vi "Dashboard Main.vi"() -> ()   [LabVIEW 2011]
uses:
  Dashboard Datatype.ctl
  <vilib>/Rock Robotics/WPI/DriverStation/WPI_DriverStationDigitalData.ctl
  <vilib>/vision/NI_Vision_Development_Module.lvlib
panel:
  out "Bounding Box":T1
  out "TargetDistance":dbl
  out "Camera Image 2":T2(plugin-control) caption="Zoomed Image"
  out "Odometer":dbl
  out "Encoders":cluster{"Left Encoder":dbl, "Right Encoder":dbl}
  out "Launcher Rate":dbl
  out "Gyro":cluster{"Robot Gyro":dbl, "Robot Gyro":dbl}(knob) scale=-180.0..180.0
  out "8 -- Battery":sgl(graph)
  out "Analog Input":sgl[](array[slide]) scale=0.0..5.0
  in  "Viewer":enum32{"Camera Image", "Kinect Skeleton"}(tab)
  in  "Video Enable":bool=TRUE
  out "Camera Image":T2(plugin-control)
  out "Buttons 1":cluster{"1":bool, "2":bool, "3":bool}
  out "Kinect 1":cluster{"X":dbl, "Y":dbl, "Z":dbl} {"X" scale=1.0..-1.0; "Y" scale=1.0..-1.0; "Z" scale=1.0..-1.0}
  out "Buttons 2":cluster{"1":bool, "2":bool, "3":bool}
  out "Kinect 2":cluster{"X":dbl, "Y":dbl, "Z":dbl} {"X" scale=1.0..-1.0; "Y" scale=1.0..-1.0; "Z" scale=1.0..-1.0}
  out "Version":string
  out "Skeleton Picture":picture
  out "Players":i8
  out "Dashboard Datatype Warning":string="Warning: The Dashboard Datatype used by the robot project and this dashboard do not match.\nSee diagram for more details."
  out "Robot IP Address":string
  out "Image Error Message":string="Timeout in Camera Communications"
  out "Solenoid Output":bool[](array[boolean])
  out "PWM":cluster{u8, u8}[](array[slide])=[{0, 157}, {0, 157}, {0, 157}, {0, 157}, {0, 157}, {0, 157}, {0, 157}, {0, 157}, {0, 157}, {0, 169}] scale=1.0..255.0
  out "GPIO Output Enable":bool[](array[boolean])
  out "GPIO State":bool[](array[boolean])
  out "Relay":cluster{"Forward":bool[], "Reverse":bool[]}
  # "Analog #1"
  # "1"
  # "7"
  # "Communications"
  # "Solenoid #1"
  # "1"
  # "8"
  # "Digital #1"
  # "1"
  # "10"
  # "1"
  # "14"
  # "1"
  # "8"
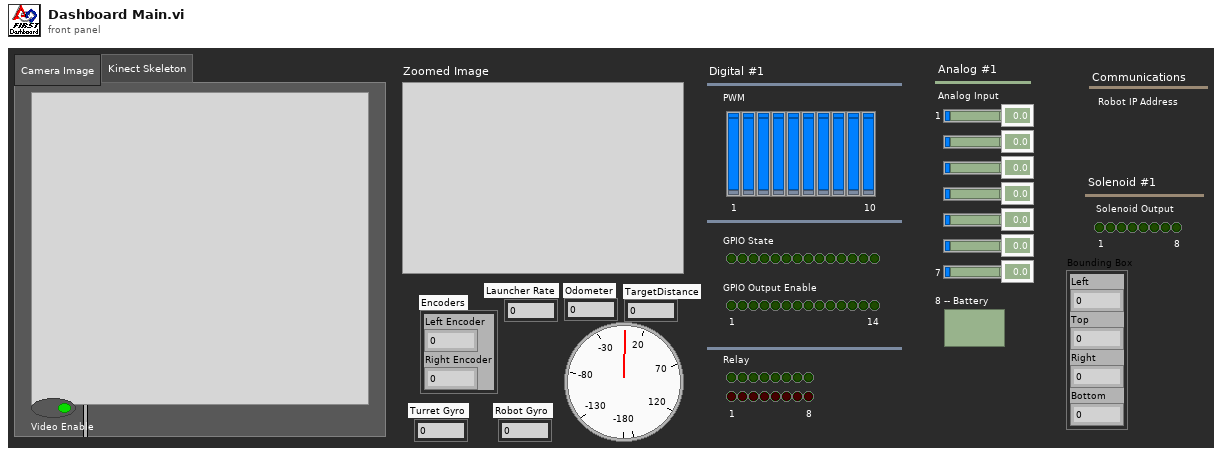
[diagram p1: front panel]
types:
  T1 = cluster{"Left":dbl, "Top":dbl, "Right":dbl, "Bottom":dbl}
  T2 = typedef "IMAQ Image.ctl" = refnum<image>
  T3 = typedef "Image Type" = u32
  T4 = typedef "Dashboard Datatype.ctl" = cluster{cluster{"AnalogModule[0]":cluster{"Channel[0]":sgl, "Channel[1]":sgl, "Channel[2]":sgl, "Channel[3]":sgl, "Channel[4]":sgl, "Channel[5]":sgl, "Channel[6]":sgl, "Channel[7]":sgl}, "AnalogModule[1]":cluster{"Channel[0]":sgl, "Channel[1]":sgl, "Channel[2]":sgl, "Channel[3]":sgl, "Channel[4]":sgl, "Channel[5]":sgl, "Channel[6]":sgl, "Channel[7]":sgl}}, cluster{"DigitalModule[0]":T5, "DigitalModule[1]":T5}, "Solenoid":u8, "Launcher Rate":dbl, "Gyros":cluster{"Turret Gyro":dbl, "Robot Gyro":dbl}, "Encoders":cluster{"Left Encoder":dbl, "Right Encoder":dbl}, "Drive Distance":dbl, "Bounding Box":cluster{"Left":dbl, "Top":dbl, "Right":dbl, "Bottom":dbl}, "Target Distance":dbl}
  T5 = typedef "WPI_DriverStationDigitalData.ctl" = cluster{"Relay Fwd":u8, "Relay Rev":u8, "GPIO":u16, "GPIO_OE":u16, "PWM":cluster{"PWM[0]":u8, "PWM[1]":u8, "PWM[2]":u8, "PWM[3]":u8, "PWM[4]":u8, "PWM[5]":u8, "PWM[6]":u8, "PWM[7]":u8, "PWM[8]":u8, "PWM[9]":u8}}
  T6 = cluster{cluster{"Left":dbl, "Bottom":dbl}, cluster{"Right":dbl, "Bottom":dbl}, cluster{"Right":dbl, "Top":dbl}, cluster{"Left":dbl, "Top":dbl}}
  T7 = typedef "LVRectTypeDef.ctl" = cluster{"left":i16, "top":i16, "right":i16, "bottom":i16}
  T8 = typedef "SkeletonTrackState.ctl" = enum32{"NotTracked", "PositionOnly", "Tracked"}
  T9 = cluster{"TrackingState":u8[], "Position":cluster{"x":sgl, "y":sgl, "z":sgl}, cluster{"x":sgl, "y":sgl, "z":sgl, sgl}[], "TrackState":T8}
  T10 = cluster{cluster{"ScaledToPercentRange":dbl, "ScaledToPercentRange":dbl, "ScaledToPercentRange":dbl}, cluster{bool, bool, bool}}[]
  T11 = typedef "LVBoundsTypeDef.ctl" = cluster{"Width":u32, "Height":u32}
  T12 = cluster{cluster{"ScaledToPercentRange":dbl, "ScaledToPercentRange":dbl, "ScaledToPercentRange":dbl}, cluster{bool, bool, bool}}
  T13 = cluster{"ScaledToPercentRange":dbl, "ScaledToPercentRange":dbl, "ScaledToPercentRange":dbl}
  T14 = cluster{"Competition mode":bool, "Robot Link":bool, "Autonomous":bool, "Enabled":bool, "E-Stop":bool}
  T15 = cluster{"AnalogModule[0]":cluster{"Channel[0]":sgl, "Channel[1]":sgl, "Channel[2]":sgl, "Channel[3]":sgl, "Channel[4]":sgl, "Channel[5]":sgl, "Channel[6]":sgl, "Channel[7]":sgl}, "AnalogModule[1]":cluster{"Channel[0]":sgl, "Channel[1]":sgl, "Channel[2]":sgl, "Channel[3]":sgl, "Channel[4]":sgl, "Channel[5]":sgl, "Channel[6]":sgl, "Channel[7]":sgl}}
  T16 = cluster{"DigitalModule[0]":T5, "DigitalModule[1]":T5}
  T17 = cluster{"Channel[0]":sgl, "Channel[1]":sgl, "Channel[2]":sgl, "Channel[3]":sgl, "Channel[4]":sgl, "Channel[5]":sgl, "Channel[6]":sgl, "Channel[7]":sgl}[]
  T18 = cluster{"Channel[0]":sgl, "Channel[1]":sgl, "Channel[2]":sgl, "Channel[3]":sgl, "Channel[4]":sgl, "Channel[5]":sgl, "Channel[6]":sgl, "Channel[7]":sgl}
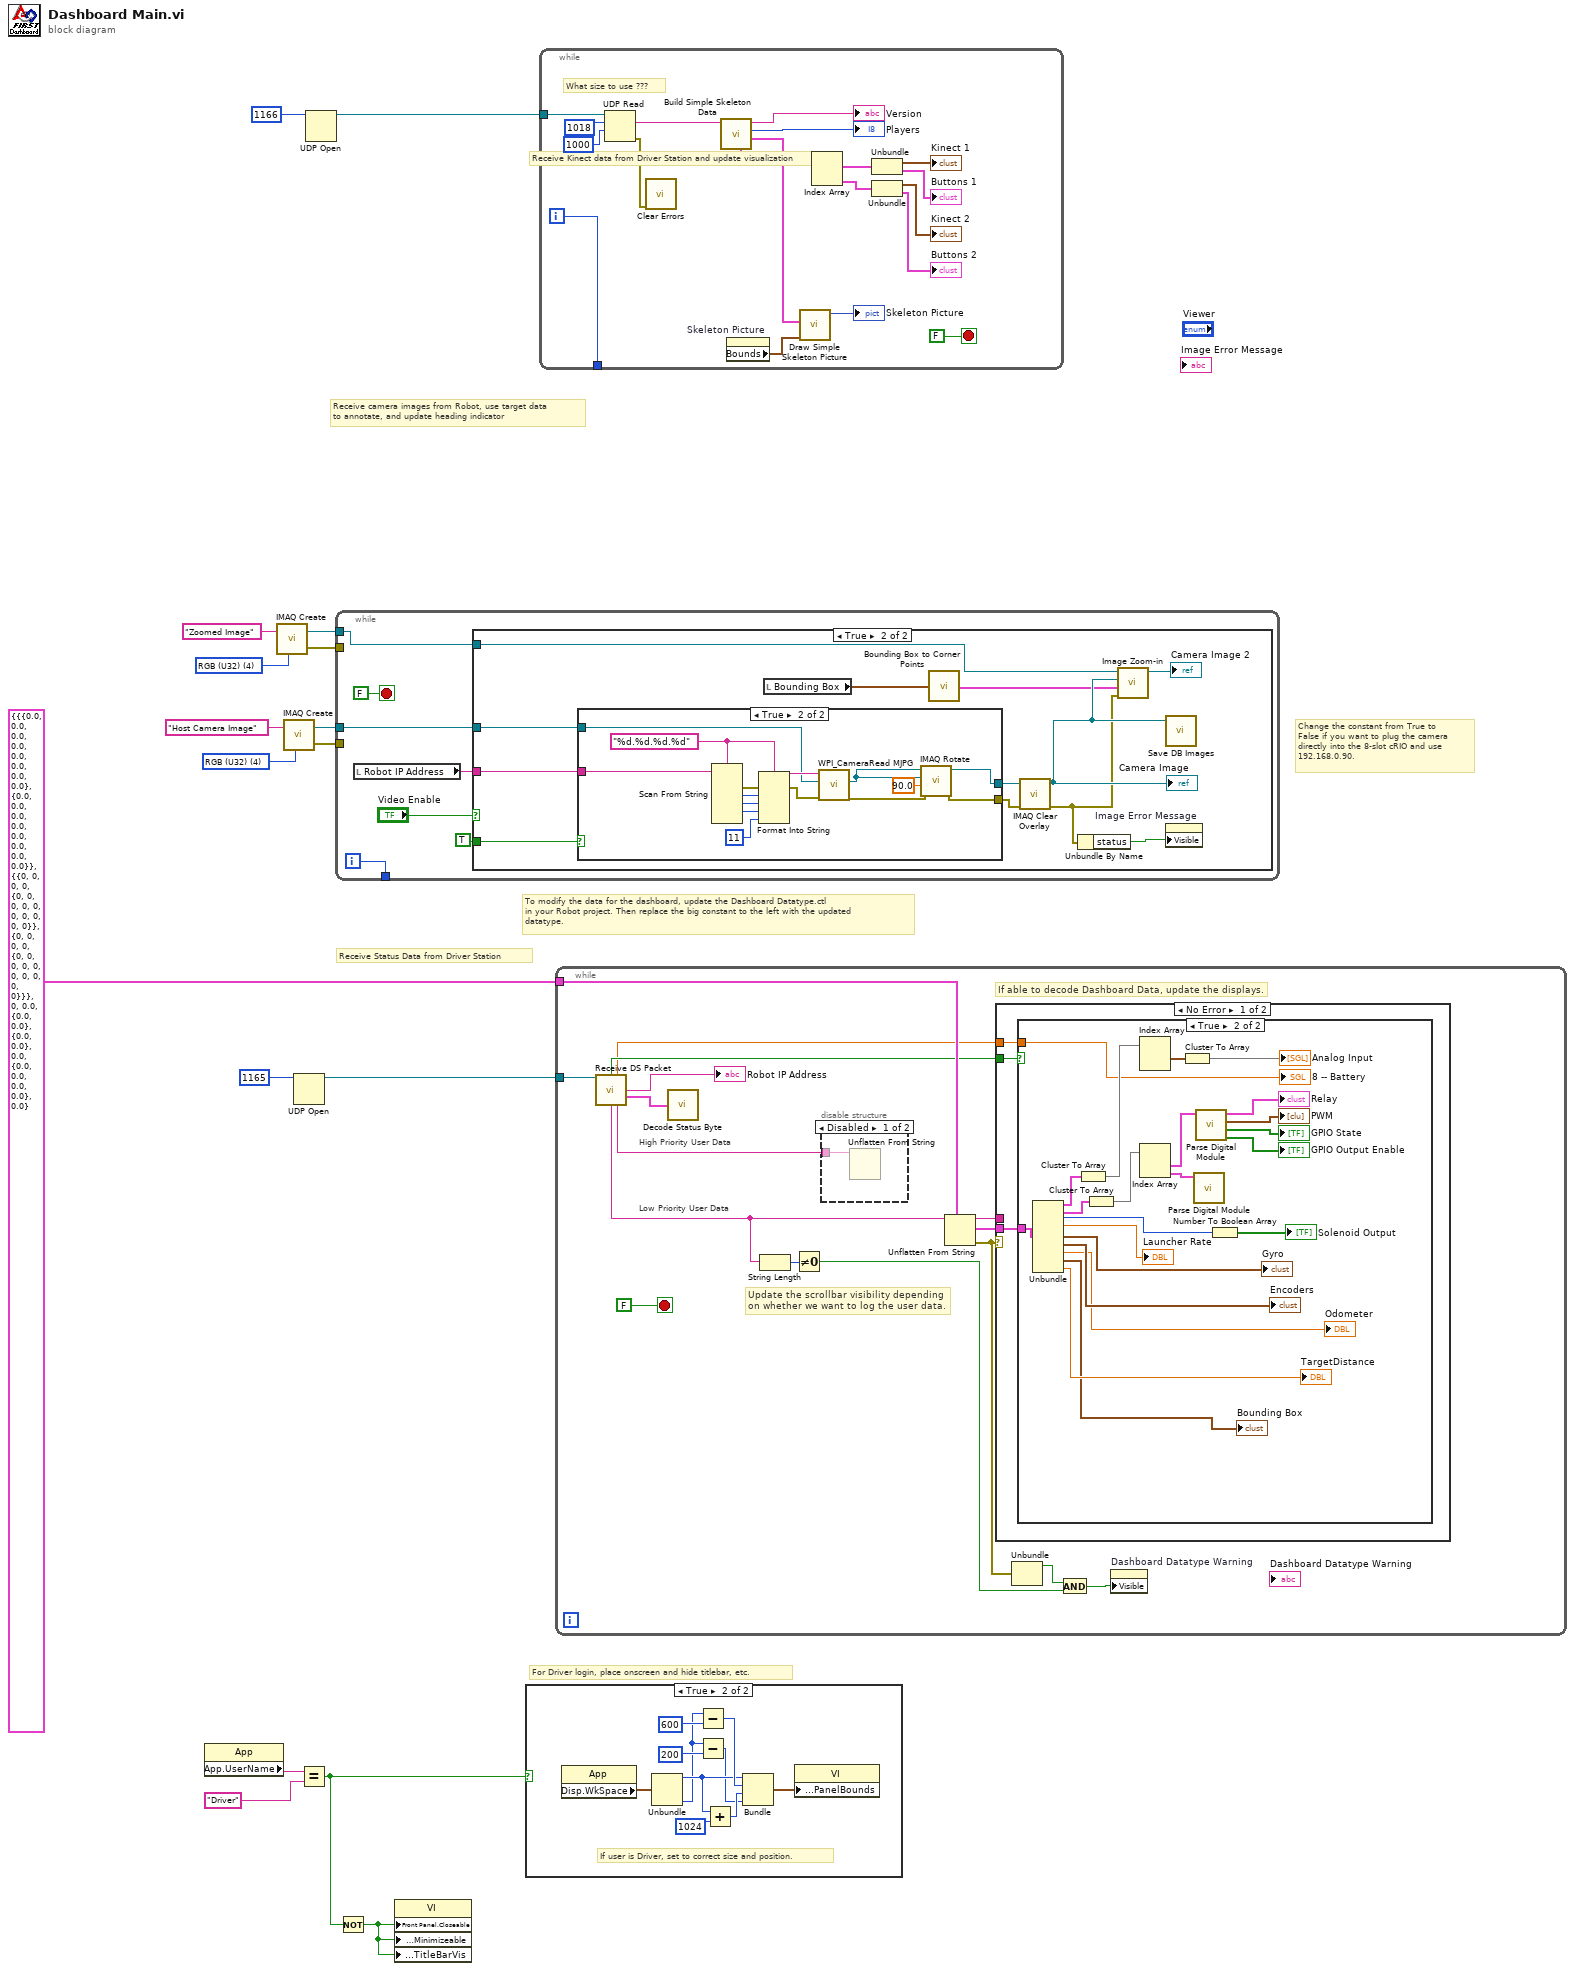
[diagram p0: block diagram]
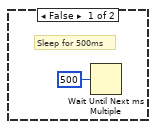
[diagram p6: hidden frame]
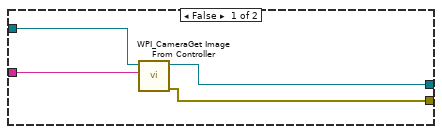
[diagram p7: hidden frame]
diagram:
  w4 = T3 4 items=["Grayscale (U8)", "Grayscale (I16)", "Grayscale (SGL)", "Complex (CSG)", "RGB (U32)", "HSL (U32)", "RGB (U64)"] ("Image Type")
  w15 = T3 4 items=["Grayscale (U8)", "Grayscale (I16)", "Grayscale (SGL)", "Complex (CSG)", "RGB (U32)", "HSL (U32)", "RGB (U64)"] ("Image Type")
  # "Change the constant from True to\nFalse if you want to plug the camera\ndirectly into the 8-slot cRIO and use\n192.168.0.90."
  # "Receive Kinect data from Driver Station and update visualization"
  # "For Driver login, place onscreen and hide titlebar, etc."
  # "To modify the data for the dashboard, update the Dashboard Datatype.ctl\nin your Robot project. Then replace the big constant to the left with the updated\ndatatype."
  # "Receive Status Data from Driver Station"
  # "Receive camera images from Robot, use target data\nto annotate, and update heading indicator"
  n1 = property class="App"() -> ("App.UserName"=w10:string)  [unwired: 2 in, 2 out]
  n2 = call "IMAQ Create"("Image Name"="Zoomed Image", "Image Type"=w4) -> ("New Image"=w2:T2, "error out"=w1:errorcluster)  [unwired: 2 in, 1 out]
  n3 = call "IMAQ Create"("Image Name"="Host Camera Image", "Image Type"=w15) -> ("New Image"=w13:T2, "error out"=w12:errorcluster)  [unwired: 2 in, 1 out]
  n4 = UDP Open(11:u16 1165 ("port")) -> (port=w16:refnum<k16>)  [unwired: 2 in, 4 out]
  n5 = Equal?(x=w10, y="Driver") -> (x = y?=w9:bool)
  n6 = UDP Open(11:u16 1166 ("port")) -> (port=w6:refnum<k16>)  [unwired: 2 in, 4 out]
  n7 = while {
    tunnel: w13 -> [w22]
    tunnel: w12 -> [_]
    tunnel: [w19] -> _
    tunnel: w2 -> [w18]
    tunnel: w1 -> [_]
    i -> [w19]
    stop <- FALSE stop-if-true
    n8 = local read "Robot IP Address"() -> (w23:string)
    n9 = case shown="True" "Video Enable" {
      tunnel: w23 -> [_ w37]
      tunnel: w22 -> [_ w36]
      tunnel: TRUE -> [_ w33]
      tunnel: w18 -> [_ w30]
      frame False {
        # "Sleep for 500ms"
        n10 = Wait Until Next ms Multiple(millisecond multiple=u32 500) -> ()  [unwired: 1 out]
      }
      frame True {
        n11 = case shown="True" w33 {
          tunnel: w36 -> [w40 w50]
          tunnel: [w38 w44] -> w29
          tunnel: [w39 w43] -> w34
          tunnel: w37 -> [w41 w53]
          frame False {
            n12 = call <vilib>:"WPI_CameraGet Image From Controller.vi"("Controller Address"=w41, "Image"=w40) -> ("error out"=w38:errorcluster, "Image Out"=w39:T2)  [unwired: 2 in, 6 out]
          }
          frame True {
            w42 = "%d.%d.%d.%d" ("format string")
            n13 = Scan From String(format string=w42, input string=w53) -> (error out=w52:errorcluster, output 1=w54:i32, output 2=w55:i32, output 3=w56:i32)  [unwired: 2 in, 7 out]
            n14 = Format Into String(format string=w42, error in=w52, w54, w55, w56, 11 ("IP Suffix:")) -> (resulting string=w51:string, error out=w49:errorcluster)  [unwired: 1 in]
            n15 = call <vilib>:"WPI_CameraRead MJPG.vi"("error in"=w49, "Image"=w50, "address"=w51) -> ("error out"=w45:errorcluster, "Image Out"=w46:T2)  [unwired: 7 in]
            n16 = call "IMAQ Rotate"("error in (no error)"=w45, "Angle (degrees)"=sgl 90.0, "Image Dst"=w46, "Image Src"=w46) -> ("error out"=w44:errorcluster, "Image Dst Out"=w43:T2)  [unwired: 6 in]
          }
        }
        n17 = local read "Bounding Box"() -> (w28:T1)
        n18 = call "Bounding Box to Corner Points.vi"("Bounding Box"=w28) -> ("Rectangle Points Out"=w27:T6)
        n19 = call "IMAQ Clear Overlay"("error in (no error)"=w29, "Image"=w34) -> ("error out"=w26:errorcluster, "Image Out"=w31:T2)  [unwired: 1 in, 7 out]
        "Camera Image" <- w31
        n20 = Unbundle By Name(w26) -> ("status"=w35:bool)
        n21 = call "Image Zoom-in.vi"("error in (no error)"=w26, "Target Corners"=w27, "Original"=w31, "Processed"=w30) -> ("Processed out"=→"Camera Image 2":T2)  [unwired: 6 in, 1 out]
        n22 = call "Save DB Images.vi"("Image"=w31) -> ()  [unwired: 2 in, 1 out]
        n23 = property on="Image Error Message" class="Str"("Visible"=w35) -> ()  [unwired: 2 in, 2 out]
      }
    }
  }
  n24 = Not(x=w9) -> (.not. x?=w8:bool)
  n25 = property class="VI"("Front Panel.Closeable"=w8, "Front Panel.Minimizeable"=w8, "Front Panel.TitleBarVis"=w8) -> ()  [unwired: 2 in, 2 out]
  n26 = case shown="True" w9 {
    frame False {
    }
    frame True {
      # "If user is Driver, set to correct size and position."
      n27 = property class="App"() -> ("Disp.WkSpace"=w66:T7)  [unwired: 2 in, 2 out]
      n28 = Unbundle(w66) -> ("left"=w61:i16, "bottom"=w57:i16)  [unwired: 2 out]
      n29 = Subtract(x=w57, y=600) -> (x-y=w63:i32)
      n30 = Subtract(x=w57, y=200) -> (x-y=w58:i32)
      n31 = Add(x=w61, y=1024) -> (x+y=w62:i32)
      n32 = Bundle("left"=w61, w63, w62, w58) -> (w65:cluster{"left":i16, i32, i32, i32})  [unwired: 1 out]
      n33 = property class="VI"("Front Panel.PanelBounds"=w65) -> ()  [unwired: 2 in, 2 out]
    }
  }
  n34 = while {
    tunnel: w6 -> [w83]
    tunnel: [w67] -> _
    i -> [w67]
    stop <- FALSE stop-if-true
    # "What size to use ???"
    n35 = UDP Read(connection ID=w83, max size (548)=1018 ("bytes to read"), timeout ms (25000)=1000) -> (data out=w77:string, error out=w75:errorcluster)  [unwired: 1 in, 3 out]
    n36 = call <vilib>:"Clear Errors.vi"("error in (no error)"=w75) -> ()  [unwired: 6 in, 1 out]
    n37 = call "Build Simple Skeleton Data.vi"("data out"=w77) -> ("Skeleton Data"=w78:T9, "NumPlayers"=→"Players":i8, "Version String"=→"Version":string, "Simple Joystick Info"=w74:T10)  [unwired: 6 in, 1 out]
    n38 = property on="Skeleton Picture" class="Pict"() -> ("Bounds"=w79:T11)  [unwired: 2 in, 2 out]
    n39 = call "Draw Simple Skeleton Picture.vi"("Bounds"=w79, "Simple Skeleton"=w78) -> ("new picture out"=→"Skeleton Picture":picture)  [unwired: 9 in]
    n40 = Index Array(array=w74) -> (element #1=w73:T12, element #2=w72:T12)  [unwired: 2 in]
    n41 = Unbundle(w73) -> (→"Kinect 1":T13, →"Buttons 1":cluster{bool, bool, bool})
    n42 = Unbundle(w72) -> (→"Kinect 2":T13, →"Buttons 2":cluster{bool, bool, bool})
  }
  n43 = while {
    tunnel: w16 -> [w99]
    tunnel: T4 {{"AnalogModule[0]"={"Channel[0]"=0.0, "Channel[1]"=0.0, "Channel[2]"=0.0, "Channel[3]"=0.0, "Channel[4]"=0.0, "Channel[5]"=0.0, "Channel[6]"=0.0, "Channel[7]"=0.0}, "AnalogModule[1]"={"Channel[0]"=0.0, "Channel[1]"=0.0, "Channel[2]"=0.0, "Channel[3]"=0.0, "Channel[4]"=0.0, "Channel[5]"=0.0, "Channel[6]"=0.0, "Channel[7]"=0.0}}, {"DigitalModule[0]"={"Relay Fwd"=0, "Relay Rev"=0, "GPIO"=0, "GPIO_OE"=0, "PWM"={"PWM[0]"=0, "PWM[1]"=0, "PWM[2]"=0, "PWM[3]"=0, "PWM[4]"=0, "PWM[5]"=0, "PWM[6]"=0, "PWM[7]"=0, "PWM[8]"=0, "PWM[9]"=0}}, "DigitalModule[1]"={"Relay Fwd"=0, "Relay Rev"=0, "GPIO"=0, "GPIO_OE"=0, "PWM"={"PWM[0]"=0, "PWM[1]"=0, "PWM[2]"=0, "PWM[3]"=0, "PWM[4]"=0, "PWM[5]"=0, "PWM[6]"=0, "PWM[7]"=0, "PWM[8]"=0, "PWM[9]"=0}}}, "Solenoid"=0, "Launcher Rate"=0.0, "Gyros"={"Turret Gyro"=0.0, "Robot Gyro"=0.0}, "Encoders"={"Left Encoder"=0.0, "Right Encoder"=0.0}, "Drive Distance"=0.0, "Bounding Box"={"Left"=0.0, "Top"=0.0, "Right"=0.0, "Bottom"=0.0}, "Target Distance"=0.0} ("Dashboard Data") -> [w98]
    stop <- FALSE stop-if-true
    # "High Priority User Data"
    # "Low Priority User Data"
    # "Update the scrollbar visibility depending\non whether we want to log the user data."
    # "If able to decode Dashboard Data, update the displays."
    n44 = call "Receive DS Packet.vi"("Recv Socket"=w99) -> ("New Dashboard Data"=w95:bool, "Battery"=w86:sgl, "Robot IP Address"=→"Robot IP Address":string, "Status"=w100:T14, "Low Priority User Data"=w88:string, "High Priority User Data"=w87:string)  [unwired: 1 in, 8 out]
    n45 = call "Decode Status Byte.vi"("Status Byte"=w100) -> ()  [unwired: 2 out]
    n46 = String Length(string=w88) -> (length=w90:i32)
    n47 = Not Equal To 0?(x=w90) -> (x != 0?=w93:bool)
    n48 = disable-structure shown="Disabled" {
      disable-tunnel: w87 -> [w102 _]
      frame Disabled {
        n49 = Unflatten From String(binary string=w102) -> ()  [unwired: 2 in, 5 out]
      }
      frame Enabled {
      }
    }
    n50 = Unflatten From String(type=w98, binary string=w88) -> (rest of the binary string=w91:string, value=w97:T4, error out=w96:errorcluster)  [unwired: 1 in, 2 out]
    n51 = case shown="No Error" w96 {
      tunnel: w97 -> [w105 _]
      tunnel: w95 -> [w104 _]
      tunnel: w91 -> [_ _]
      tunnel: w86 -> [w103 _]
      frame No Error {
        n52 = case shown="True" w104 {
          tunnel: w105 -> [_ w118]
          tunnel: w103 -> [_ w112]
          frame False {
            # "Don't update if the robot hasn't sent new data"
          }
          frame True {
            n53 = Unbundle(w118) -> (w115:T15, w116:T16, "Solenoid"=w117:u8, "Launcher Rate"=→"Launcher Rate":dbl, "Gyros"=→"Gyro":cluster{"Turret Gyro":dbl, "Robot Gyro":dbl}, "Encoders"=→"Encoders":cluster{"Left Encoder":dbl, "Right Encoder":dbl}, "Drive Distance"=→"Odometer":dbl, "Bounding Box"=→"Bounding Box":T1, "Target Distance"=→"TargetDistance":dbl)
            n54 = Cluster To Array(cluster=w115) -> (array=w126:T17)
            n55 = Cluster To Array(cluster=w116) -> (array=w125:T5[])
            n56 = Index Array(array=w126) -> (element #1=w113:T18)  [unwired: 2 in, 1 out]
            n57 = Index Array(array=w125) -> (element #1=w124:T5, element #2=w119:T5)  [unwired: 2 in]
            n58 = Cluster To Array(cluster=w113) -> (array=→"Analog Input":sgl[])
            n59 = call "Parse Digital Module.vi"("DigitalModule"=w119) -> ()  [unwired: 11 out]
            n60 = call "Parse Digital Module.vi"("DigitalModule"=w124) -> ("GPIO Output Enable"=→"GPIO Output Enable":bool[], "GPIO State"=→"GPIO State":bool[], "PWM"=→"PWM":cluster{u8, u8}[], "Relay"=→"Relay":cluster{"Forward":bool[], "Reverse":bool[]})  [unwired: 7 out]
            n61 = Number To Boolean Array(number=w117) -> (Boolean array=→"Solenoid Output":bool[])
            "8 -- Battery" <- w112
          }
        }
      }
      frame Error {
        # "Your datatypes don't match. The Dashboard Datatype.ctl in your Robot project\nand the big constant to the left of the loop need to match."
      }
    }
    n62 = Unbundle(w96) -> ("status"=w92:bool)  [unwired: 2 out]
    n63 = And(x=w92, y=w93) -> (x .and. y?=w94:bool)
    n64 = property on="Dashboard Datatype Warning" class="Str"("Visible"=w94) -> ()  [unwired: 2 in, 2 out]
  }
